vi "ROE200_Driver.vi"(0 "STATUS INPUT":T1(ring)=enum."HOMING", 1 "VISA resource name":refnum<visa-resource-name>, 5 "X 2":u32, 7 "Y 2":u32, 9 "Z 2":u32, 11 "Timing":u32, 12 "error in (no error) 2":errorcluster) -> (3 "VISA resource name out":refnum<visa-resource-name>, 4 "STATUS OUTPUT":T1(ring)=enum."HOMING", 6 "X Position":u32, 10 "Y Position":u32, 14 "error out 2":errorcluster, 15 "Z Position":u32)   [LabVIEW 2019]
panel:
  in  "Hard Stop":u32
  out "Active Drive":i8
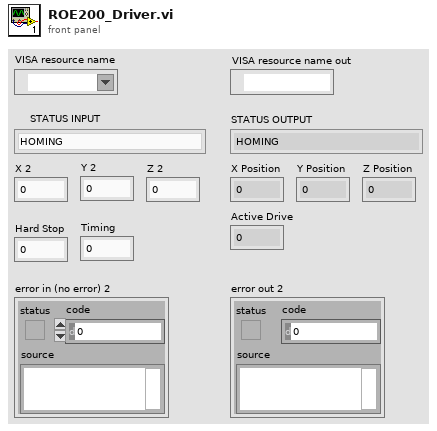
[diagram p1: front panel]
types:
  T1 = enum16{"READY", "ABSOLUTE MOVE", "RELATIVE MOVE", "HOMING", "WAITING", "CANCELING"}
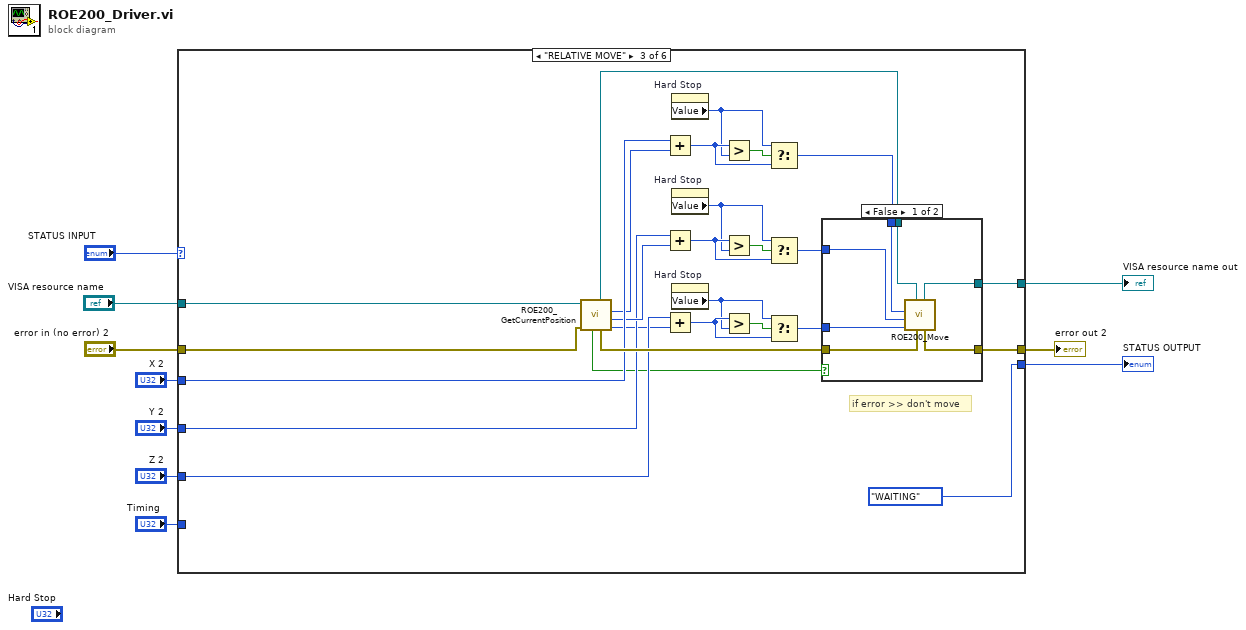
[diagram p0: block diagram]
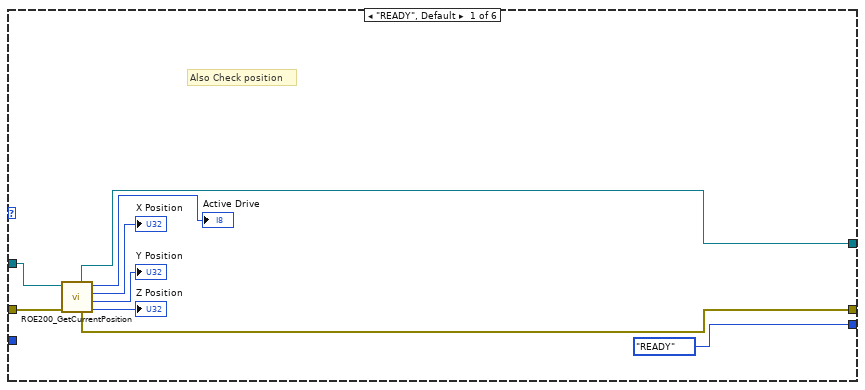
[diagram p2: hidden frame]
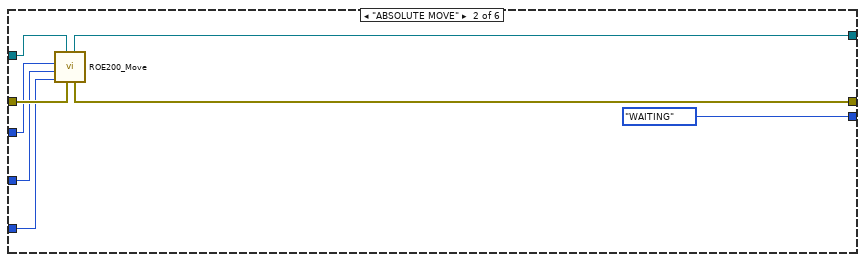
[diagram p3: hidden frame]
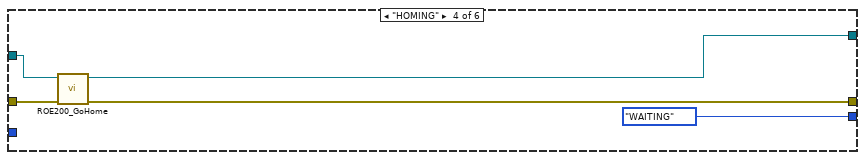
[diagram p5: hidden frame]
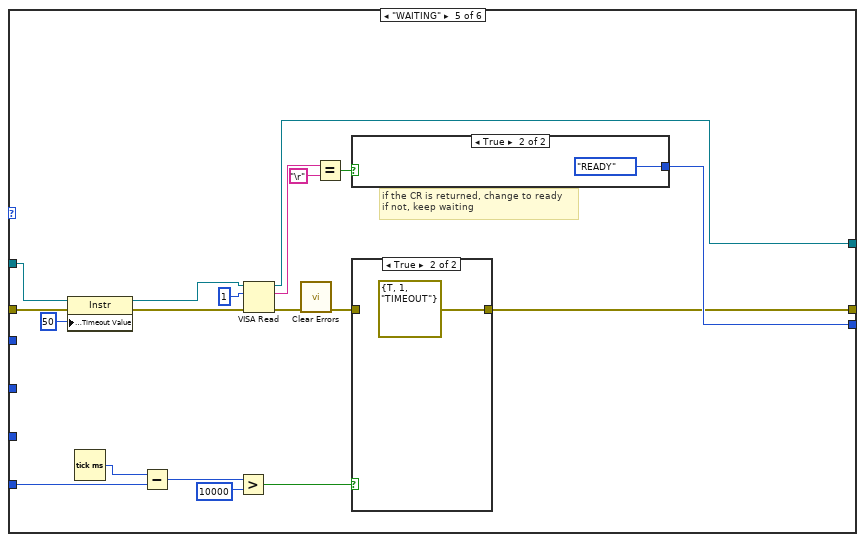
[diagram p6: hidden frame]
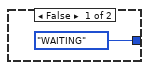
[diagram p8: hidden frame]
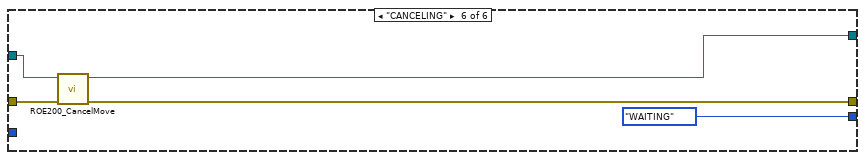
[diagram p9: hidden frame]
diagram:
  n1 = case shown="\"RELATIVE MOVE\"" "STATUS INPUT" {
    tunnel: [w17 w25 w52 w65 w68 w95] -> w10
    tunnel: "VISA resource name" -> [w19 w27 w51 w67 w78 w94]
    tunnel: [w16 w24 w53 w66 w85 w93] -> w8
    tunnel: "error in (no error) 2" -> [w18 w26 w49 w64 w77 w92]
    tunnel: [T1."READY" ("STATUS INPUT 2") T1."WAITING" ("STATUS INPUT 2") T1."WAITING" ("STATUS INPUT 2") T1."WAITING" ("STATUS INPUT 2") w86 T1."WAITING" ("STATUS INPUT 2")] -> w6
    tunnel: "X 2" -> [_ w22 w47 _ _ _]
    tunnel: "Z 2" -> [_ w21 w43 _ _ _]
    tunnel: "Y 2" -> [_ w20 w44 _ _ _]
    tunnel: "Timing" -> [_ _ _ _ w73 _]
    frame "READY", Default {
      # "Also Check position"
      n2 = call "ROE200_GetCurrentPosition.vi"("error in (no error)"=w18, "VISA resource name"=w19) -> ("Z Position"=→"Z Position":u32, "Y Position"=→"Y Position":u32, "X Position"=→"X Position":u32, "Active Drive"=→"Active Drive":u8, "error out"=w17:errorcluster, "VISA resource  out"=w16:refnum<visa-resource-name>)  [unwired: 3 in, 1 out]
    }
    frame "ABSOLUTE MOVE" {
      n3 = call "ROE200_Move.vi"("error in (no error)"=w26, "VISA resource name 2"=w27, "Z"=w21, "Y"=w20, "X"=w22) -> ("error out"=w25:errorcluster, "VISA resource name out"=w24:refnum<visa-resource-name>)  [unwired: 5 in]
    }
    frame "RELATIVE MOVE" {
      # "if error >> don't move"
      n4 = call "ROE200_GetCurrentPosition.vi"("error in (no error)"=w49, "VISA resource name"=w51) -> ("Z Position"=w42:u32, "Y Position"=w45:u32, "X Position"=w46:u32, "error out"=w48:errorcluster, "VISA resource  out"=w50:refnum<visa-resource-name>, "error in GetCurrentPosition"=w29:bool)  [unwired: 3 in, 1 out]
      n5 = Add(x=w47, y=w46) -> (x+y=w40:u32)
      n6 = Add(x=w44, y=w45) -> (x+y=w36:u32)
      n7 = Add(x=w43, y=w42) -> (x+y=w33:u32)
      n8 = property on="Hard Stop" class="DigNum (strict)"() -> ("Value"=w38:u32)  [unwired: 2 in, 2 out]
      n9 = property on="Hard Stop" class="DigNum (strict)"() -> ("Value"=w35:u32)  [unwired: 2 in, 2 out]
      n10 = property on="Hard Stop" class="DigNum (strict)"() -> ("Value"=w32:u32)  [unwired: 2 in, 2 out]
      n11 = Greater?(x=w40, y=w38) -> (0:w41:bool)
      n12 = Greater?(x=w36, y=w35) -> (0:w37:bool)
      n13 = Greater?(x=w33, y=w32) -> (0:w34:bool)
      n14 = Select(t=w38, s=w41, f=w40) -> (s? t:f=w39:u32)
      n15 = Select(t=w35, s=w37, f=w36) -> (s? t:f=w30:u32)
      n16 = Select(t=w32, s=w34, f=w33) -> (s? t:f=w31:u32)
      n17 = case shown="False" w29 {
        tunnel: [w60 w62] -> w53
        tunnel: [w59 w61] -> w52
        tunnel: w50 -> [w58 w62]
        tunnel: w48 -> [w57 w61]
        tunnel: w39 -> [w56 _]
        tunnel: w31 -> [w55 _]
        tunnel: w30 -> [w54 _]
        frame False {
          n18 = call "ROE200_Move.vi"("error in (no error)"=w57, "VISA resource name 2"=w58, "Z"=w55, "Y"=w54, "X"=w56) -> ("error out"=w59:errorcluster, "VISA resource name out"=w60:refnum<visa-resource-name>)  [unwired: 5 in]
        }
        frame True {
        }
      }
    }
    frame "HOMING" {
      n19 = call "ROE200_GoHome.vi"("error in (no error)"=w64, "VISA resource name"=w67) -> ("error out"=w65:errorcluster, "VISA resource name out"=w66:refnum<visa-resource-name>)  [unwired: 8 in]
    }
    frame "WAITING" {
      # "if the CR is returned, change to ready\nif not, keep waiting"
      n20 = property class="Instr"(reference=w78, error in=w77, "General Settings:Timeout Value"=u32 50) -> (reference out=w76:refnum<visa-resource-name>, error out=w75:errorcluster)
      n21 = Tick Count (ms)() -> (millisecond timer value=w74:u32)
      n22 = Subtract(x=w74, y=w73) -> (x-y=w72:u32)
      n23 = Greater?(x=w72, y=u32 10000) -> (0:w70:bool)
      n24 = VISA Read(VISA resource name=w76, byte count=u32 1, error in (no error)=w75) -> (VISA resource name out=w85:refnum<visa-resource-name>, read buffer=w82:string, error out=w84:errorcluster)  [unwired: 1 out]
      n25 = call <vilib>:"Clear Errors.vi"("error in (no error)"=w84) -> ("error out"=w69:errorcluster)  [unwired: 5 in, 1 out]
      n26 = Equal?(x=w82, y="\r") -> (x = y?=w83:bool)
      n27 = case shown="True" w83 {
        tunnel: [T1."WAITING" ("STATUS INPUT 2") T1."READY" ("STATUS INPUT 2")] -> w86
        frame False {
        }
        frame True {
        }
      }
      n28 = case shown="True" w70 {
        tunnel: w69 -> [w87 _]
        tunnel: [w87 errorcluster {"status"=TRUE, "code"=1, "source"="TIMEOUT"} ("error out")] -> w68
        frame False {
        }
        frame True {
        }
      }
    }
    frame "CANCELING" {
      n29 = call "ROE200_CancelMove.vi"("error in (no error)"=w92, "VISA resource name"=w94) -> ("error out"=w95:errorcluster, "VISA resource name out"=w93:refnum<visa-resource-name>)  [unwired: 8 in]
    }
  }
  "error out 2" <- w10
  "STATUS OUTPUT" <- w6
  "VISA resource name out" <- w8
